vi "MulticastAnswerTbl (SubVI).vi"(8 "count":i32, 11 "SUdpAnswer":T1) -> (3 "Array":string[](array[string]))   [LabVIEW 2017, in "LV_Unicorn.lvlib"]
uses:
  LV_Unicorn.lvlib
  Control/AnswerUDP.ctl
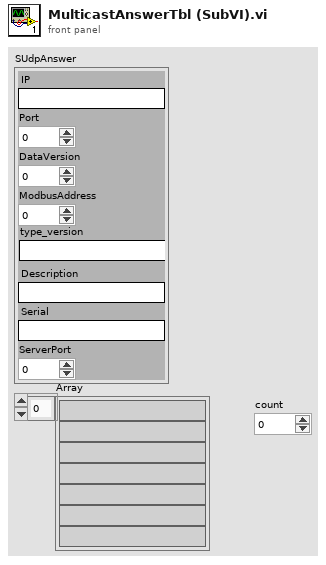
[diagram p1: front panel]
types:
  T1 = typedef "LV_Unicorn.lvlib/AnswerUDP.ctl" = cluster{"IP":string, "Port":u16, "DataVersion":u16, "ModbusAddress":i32, "type_version":string, "Description":string, "Serial":string, "ServerPort":u16}
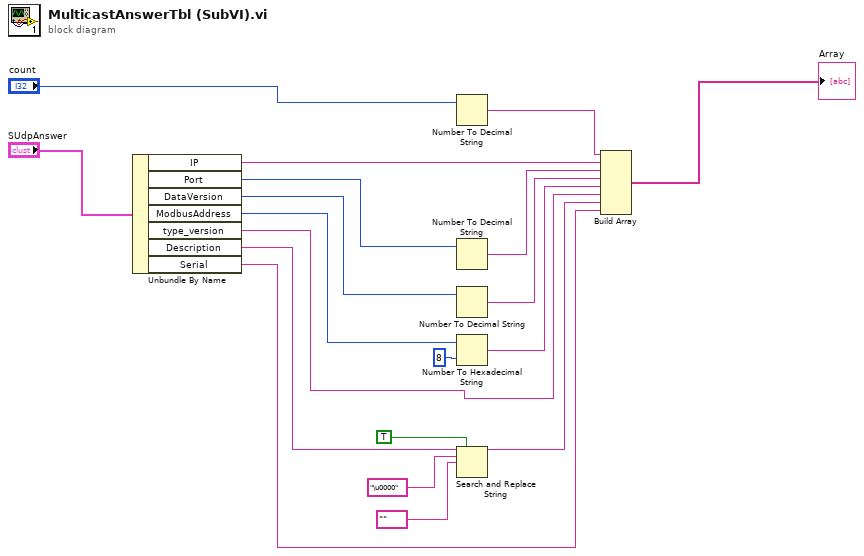
[diagram p0: block diagram]
diagram:
  n1 = Unbundle By Name("SUdpAnswer") -> ("IP"=w10:string, "Port"=w9:u16, "DataVersion"=w8:u16, "ModbusAddress"=w7:i32, "type_version"=w1:string, "Description"=w6:string, "Serial"=w5:string)
  n2 = Number To Decimal String(number="count") -> (decimal integer string=w3:string)  [unwired: 1 in]
  n3 = Number To Decimal String(number=w9) -> (decimal integer string=w16:string)  [unwired: 1 in]
  n4 = Number To Decimal String(number=w8) -> (decimal integer string=w17:string)  [unwired: 1 in]
  n5 = Number To Hexadecimal String(1:i16 8 ("width (-)"), 2:w7) -> (0:w18:string)
  n6 = Search and Replace String(replace all?=TRUE ("replace all? (F)"), input string=w6, search string="\u0000", replace string="" ("replace string (\"\")")) -> (result string=w12:string)  [unwired: 4 in, 3 out]
  n7 = Build Array(w3, w10, w16, w17, w18, w1, w12, w5) -> (→"Array":string[])
